vi "pulse_in.vi"() -> ()   [LabVIEW 2019]
uses:
  <vilib>/Platform/TimedLoop/XDataNode/timing_clust.ctl
  <vilib>/Platform/TimedLoop/XDataNode/nitl_modes.ctl
  <vilib>/Platform/TimedLoop/XDataNode/wakeup.ctl
  <vilib>/rvi/Emulation/niFpgaGetClockAttributes.vi
  <vilib>/rvi/Emulation/niFpgaSctlEmulationGetInTimedLoop.vi
  <vilib>/rvi/Emulation/niFpgaEmulationReportErrorSimple.vi
  <vilib>/rvi/Emulation/niFpgaProcessEmulError.vi
  <vilib>/rvi/eio/common/nirviEmuTemplateMethod_errors.vi
  <vilib>/rvi/Emulation/niFpgaCriticalErrorInLSC.vi
  <vilib>/eio/EIONode/EIONode.xnode
  <vilib>/Platform/TimedLoop/XDataNode/XDataNode.xnode
  <vilib>/Platform/TimedLoop/XDataNode/XDNodeRunTimeDep.lvlib
panel:
  in  "stop":bool
  out "High Period (ticks)":u32
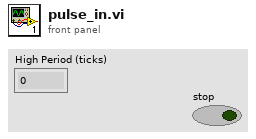
[diagram p1: front panel]
types:
  T1 = typedef "XDNodeRunTimeDep.lvlib/timing_clust.ctl" = cluster{"Expected End [f-1]":u64, "Actual End [f-1]":u64, "Finished Late? [f-1]":bool, "Expected End [i-1]":u64, "Actual End [i-1]":u64, "Finished Late? [i-1]":bool, "Expected Start [i]":u64, "Actual Start [i]":u64, "Expected Start [f]":u64, "Actual Start [f]":u64, "Source Name":string, "Structure Name":string, "Period":i64, "Deadline":i64, "Offset":i64, "Start":i64, "Priority":i32, "Timeout":i32, "Mode":T2, "Wakeup Reason":T3, "Error":errorcluster, "Source Type":string, "Secondary Source Type":string, "Global End Time":u64, "Global Start Time":u64, "Frame Duration":u64, "Iteration Duration":u64, "Assigned CPU":i32, "I/O Scan Engine Mode":u32}
  T2 = typedef "XDNodeRunTimeDep.lvlib/nitl_modes.ctl" = enum32{"No Change", "Process missed periods, maintain original phase", "Discard missed periods, maintain original phase", "Process missed periods, ignore original phase", "Discard missed periods, ignore original phase"}
  T3 = typedef "XDNodeRunTimeDep.lvlib/wakeup.ctl" = enum32{"Normal", "Aborted", "Asynchronous wakeup", "Timing source error", "Timed loop error", "Timeout"}
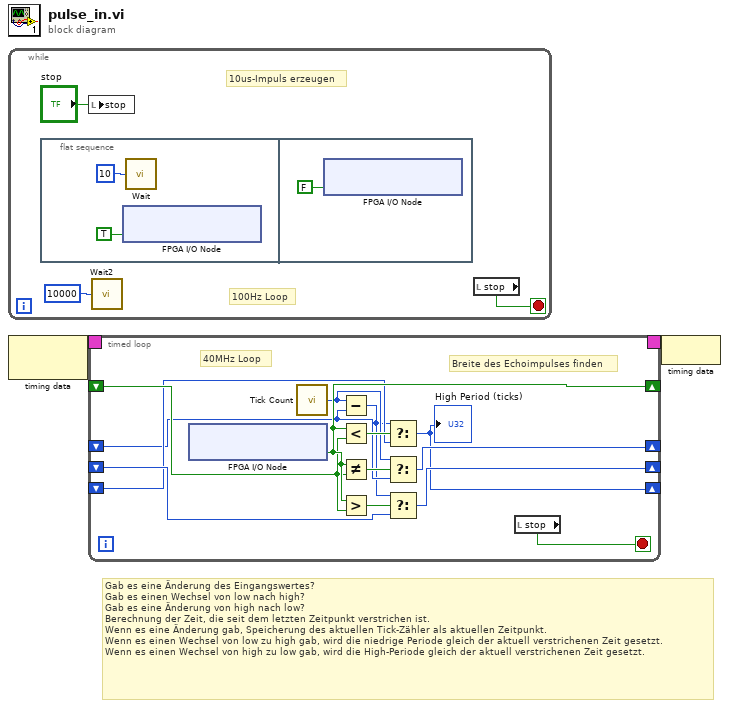
[diagram p0: block diagram]
diagram:
  # "Gab es eine Änderung des Eingangswertes?\nGab es einen Wechsel von low nach high?\nGab es eine Änderung von high nach low?\nBerechnung der Zeit, die seit dem letzten Zeitpunkt verstrichen ist.\nWenn es eine Änderung gab, Speicherung des aktuellen Tick-Zähler als aktuellen Zeitpunkt.\nWenn es einen Wechsel von low zu high gab, wird die niedrige Periode gleich der aktuell verstrichenen Zeit gesetzt. \nWenn es einen Wechsel von high zu low gab, wird die High-Periode gleich der aktuell verstrichenen Zeit gesetzt."
  n1 = while {
    stop <- w3 stop-if-true
    # "100Hz Loop"
    # "10us-Impuls erzeugen"
    n2 = flat-sequence {
      frame #0 {
        n3 = xnode "FPGA I/O Node"("ConnectorA/DIO0"=TRUE) -> ()  [unwired: 1 in, 1 out]
        n4 = call "Wait"("Count(uSec)"=u32 10) -> ()  [unwired: 1 out]
      }
      frame #1 {
        n5 = xnode "FPGA I/O Node"("ConnectorA/DIO0"=FALSE) -> ()  [unwired: 1 in, 1 out]
      }
    }
    n6 = local write "stop"("stop") -> ()
    n7 = call "Wait2"("Count(uSec)"=u32 10000) -> ()  [unwired: 1 out]
    n8 = local read "stop"() -> (w3:bool)
  }
  n9 = node-c288() -> (w2:T1)  [unwired: 1 in]
  n10 = timed-loop {
    timing: w2 -> [_]
    timing-out: [_] -> w1
    shift-right: [w21] -> _
    shift-left: _ -> [w20]
    shift-right: [w17] -> _
    shift-left: _ -> [w11]
    shift-right: [w16] -> _
    shift-left: _ -> [w14]
    shift-right: [w15] -> _
    shift-left: _ -> [w13]
    stop <- w9 stop-if-true
    # "40MHz Loop"
    # "Breite des Echoimpulses finden"
    n11 = xnode "FPGA I/O Node"() -> ("ConnectorA/DIO1"=w21:bool)  [unwired: 1 in, 1 out]
    n12 = call "Tick Count"() -> ("Tick Count(Ticks)"=w12:u32)
    n13 = Subtract(x=w12, y=w11) -> (x-y=w10:u32)
    n14 = Less?(x=w21, y=w20) -> (x < y?=w18:bool)
    n15 = Not Equal?(x=w21, y=w20) -> (x != y?=w22:bool)
    n16 = Greater?(x=w21, y=w20) -> (0:w19:bool)
    n17 = Select(t=w10, s=w18, f=w13) -> (s? t:f=w15:u32)
    "High Period (ticks)" <- w15
    n18 = Select(t=w12, s=w22, f=w11) -> (s? t:f=w17:u32)
    n19 = Select(t=w10, s=w19, f=w14) -> (s? t:f=w16:u32)
    n20 = local read "stop"() -> (w9:bool)
  }
  n21 = node-c288(w1) -> ()
